vi "PM100-Auto Range.vi"(0 "VISA in":refnum<visa-resource-name>, 7 "Power (W)":dbl, 11 "error in (no error)":errorcluster, 13 "Action":enum16{"Init", "Apply"}(ring)=enum."Apply") -> (15 "error out":errorcluster)   [LabVIEW 2015]
panel:
  out "Range":string
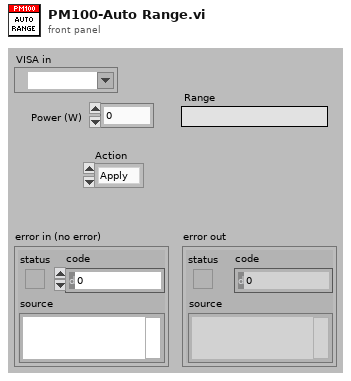
[diagram p1: front panel]
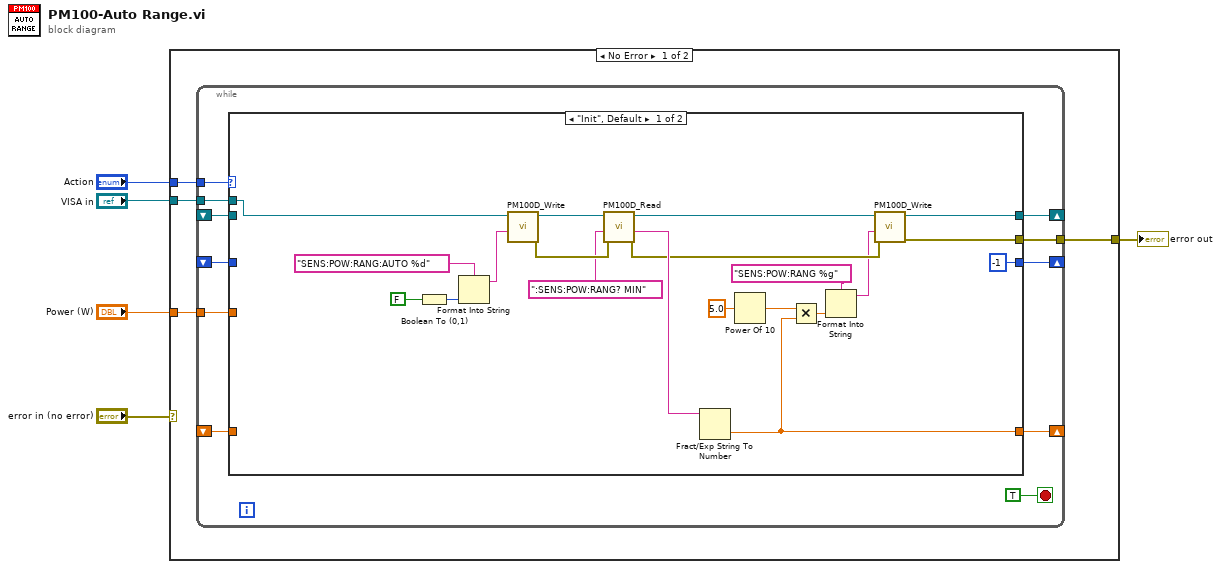
[diagram p0: block diagram]
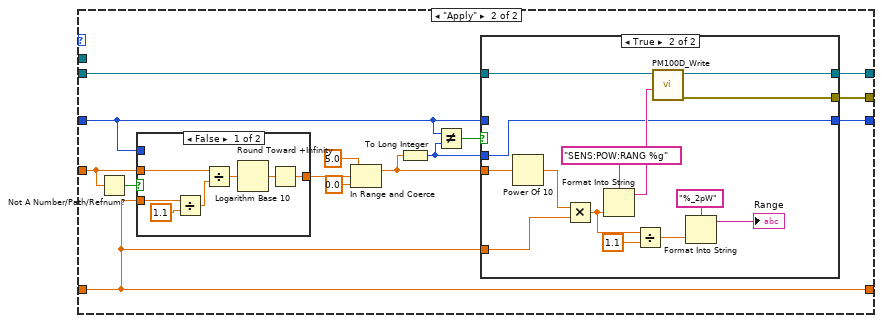
[diagram p2: hidden frame]
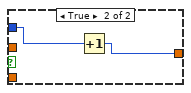
[diagram p3: hidden frame]
diagram:
  n1 = case shown="No Error" "error in (no error)" {
    selector: "error in (no error)" -> [_ w80]
    tunnel: "VISA in" -> [w7 _]
    tunnel: [w6 w80] -> w3
    tunnel: "Power (W)" -> [w9 _]
    tunnel: "Action" -> [w8 _]
    frame No Error {
      n2 = while {
        tunnel: w9 -> [w16]
        tunnel: w8 -> [w13]
        shift-right: [w17] -> _
        shift-left: _ -> [w15]
        shift-right: [w20] -> _
        shift-left: _ -> [w18]
        tunnel: w7 -> [w12]
        tunnel: [w11] -> w6
        shift-right: [w10] -> _
        shift-left: _ -> [w19]
        stop <- TRUE stop-if-true
        n3 = case shown="\"Init\", Default" w13 {
          tunnel: [w26 w54] -> w20
          tunnel: w19 -> [_ w41]
          tunnel: w18 -> [_ w51]
          tunnel: [-1 w49] -> w17
          tunnel: w16 -> [_ w48]
          tunnel: w15 -> [_ w43]
          tunnel: w12 -> [w27 _]
          tunnel: [w22 w42] -> w11
          tunnel: [w28 w41] -> w10
          frame "Init", Default {
            n4 = Boolean To (0,1)(Boolean=FALSE) -> (0, 1=w39:i16)
            n5 = Format Into String(format string="SENS:POW:RANG:AUTO %d" ("Command"), w39) -> (resulting string=w23:string)  [unwired: 2 in, 1 out]
            n6 = call "PM100D_Write.vi"("Command"=w23, "VISA in"=w27) -> ("error out"=w38:errorcluster, "VISA out"=w37:refnum<visa-resource-name>)  [unwired: 8 in]
            n7 = call "PM100D_Read.vi"("error in (no error)"=w38, "Command"=":SENS:POW:RANG? MIN", "VISA in"=w37) -> ("error out"=w30:errorcluster, "ReadValue"=w35:string, "VISA out"=w25:refnum<visa-resource-name>)  [unwired: 6 in]
            n8 = Fract/Exp String To Number(string=w35) -> (number=w28:dbl)  [unwired: 3 in, 1 out]
            n9 = Power Of 10(x=5.0) -> (10^x=w33:dbl)
            n10 = Multiply(x=w33, y=w28) -> (x*y=w31:dbl)
            n11 = Format Into String(format string="SENS:POW:RANG %g" ("Command"), w31) -> (resulting string=w21:string)  [unwired: 2 in, 1 out]
            n12 = call "PM100D_Write.vi"("error in (no error)"=w30, "Command"=w21, "VISA in"=w25) -> ("error out"=w22:errorcluster, "VISA out"=w26:refnum<visa-resource-name>)  [unwired: 7 in]
          }
          frame "Apply" {
            n13 = Not A Number/Path/Refnum?(number/path/refnum=w48) -> (NaN/Path/Refnum?=w44:bool)
            n14 = case shown="False" w44 {
              tunnel: w41 -> [w61 _]
              tunnel: w48 -> [w60 _]
              tunnel: [w55 w62] -> w47
              tunnel: w43 -> [_ w63]
              frame False {
                n15 = Divide(x=w61, y=1.1) -> (x/y=w58:dbl)
                n16 = Divide(x=w60, y=w58) -> (x/y=w59:dbl)
                n17 = Logarithm Base 10(1:w59) -> (0:w56:dbl)
                n18 = Round Toward +Infinity(x=w56) -> (ceil(x): smallest int >= x=w55:dbl)
              }
              frame True {
                n19 = Increment(x=w63) -> (x+1=w62:i32)
              }
            }
            n20 = In Range and Coerce(upper limit=5.0, x=w47, lower limit=0.0) -> (coerced(x)=w53:dbl)  [unwired: 1 out]
            n21 = To Long Integer(number=w53) -> (32bit integer=w50:i32)
            n22 = Not Equal?(x=w43, y=w50) -> (x != y?=w52:bool)
            n23 = case shown="True" w52 {
              tunnel: [w65 w78] -> w54
              tunnel: w41 -> [_ w75]
              tunnel: w53 -> [_ w74]
              tunnel: w51 -> [w65 w73]
              tunnel: w50 -> [_ w72]
              tunnel: w43 -> [w64 _]
              tunnel: [w64 w72] -> w49
              tunnel: [_ w66] -> w42
              frame False {
              }
              frame True {
                n24 = Power Of 10(x=w74) -> (10^x=w79:dbl)
                n25 = Multiply(x=w79, y=w75) -> (x*y=w71:dbl)
                n26 = Format Into String(format string="SENS:POW:RANG %g" ("Command"), w71) -> (resulting string=w76:string)  [unwired: 2 in, 1 out]
                n27 = Divide(x=w71, y=1.1) -> (x/y=w69:dbl)
                n28 = call "PM100D_Write.vi"("Command"=w76, "VISA in"=w73) -> ("error out"=w66:errorcluster, "VISA out"=w78:refnum<visa-resource-name>)  [unwired: 8 in]
                n29 = Format Into String(format string="%_2pW", w69) -> (resulting string=→"Range":string)  [unwired: 2 in, 1 out]
              }
            }
          }
        }
      }
    }
    frame Error {
    }
  }
  "error out" <- w3
